vi "Calibration Scaling (Set).vi"(6 "ISOBUS address":T4=-1 caption="ISOBUS address (-1)", 8 "error in":errorcluster, 9 "Unit":T1, 10 "Scaling Factor":dbl=0.5 min=0.5 max=1.5 step=0.1, 11 "Mercury Reference In":T5) -> (0 "error out":errorcluster, 2 "Response":T2, 3 "Mercury Reference Out":T5, 4 "Valid?":T3)   [LabVIEW 2015, in "Mercury iXX.lvlib" / "Pressure.lvlib"]
doc: "Set the current value of the pressure scaling factor."
uses:
  Pressure.lvlib
  Controls/Mercury Reference.ctl
  Controls/Comms Transport Layer.ctl
  private/Controls/Query Dynamic Reference.ctl
  Controls/ISOBus Address.ctl
  Controls/Is Valid LED.ctl
  Controls/Response String.ctl
  Controls/Unit String.ctl
  private/Controls/Command Verbs.ctl
  Mercury iXX.lvlib
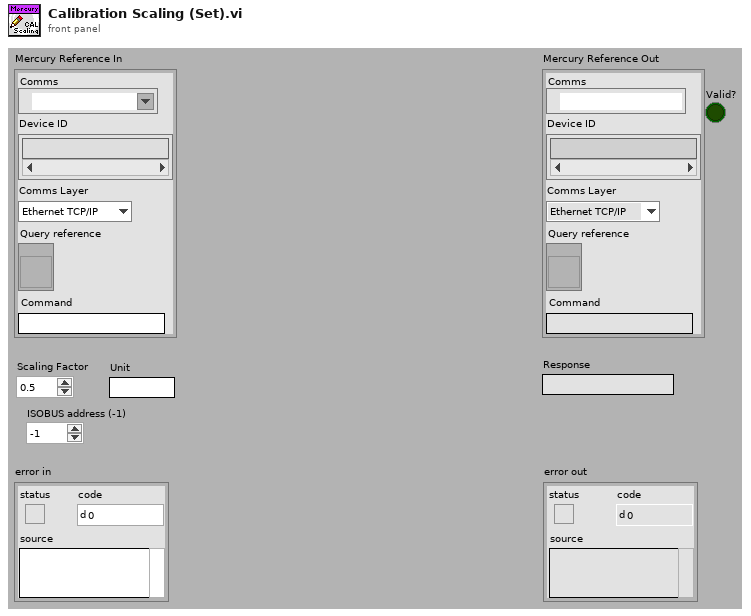
[diagram p1: front panel]
types:
  T1 = typedef "Mercury iXX.lvlib/Unit String.ctl" = string
  T2 = typedef "Mercury iXX.lvlib/Response String.ctl" = string
  T3 = typedef "Mercury iXX.lvlib/Is Valid LED.ctl" = bool
  T4 = typedef "Mercury iXX.lvlib/ISOBus Address.ctl" = i32
  T5 = typedef "Mercury iXX.lvlib/Mercury Reference.ctl" = cluster{"Comms":refnum<visa-resource-name>, "Device ID":string[], "Comms Layer":T6, "Command":string, "Query reference":T7}
  T6 = typedef "Mercury iXX.lvlib/Comms Transport Layer.ctl" = enum16{"Ethernet TCP/IP", "USB", "ISOBus - RS-232", "GPIB"}
  T7 = typedef "Mercury iXX.lvlib/Query Dynamic Reference.ctl" = refnum<vi>
  T8 = typedef "Mercury iXX.lvlib/Command Verbs.ctl" = string
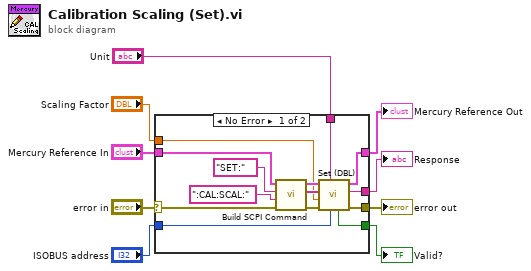
[diagram p0: block diagram]
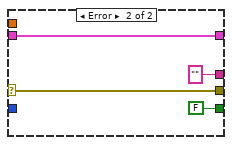
[diagram p2: hidden frame]
diagram:
  n1 = case shown="No Error" "error in" {
    selector: "error in" -> [w11 w27]
    tunnel: "Mercury Reference In" -> [w18 w26]
    tunnel: "Scaling Factor" -> [w17 _]
    tunnel: [w16 w26] -> w7
    tunnel: [w15 T2 "" ("Response")] -> w6
    tunnel: [w14 T3 FALSE ("Valid?")] -> w5
    tunnel: [w13 w27] -> w4
    tunnel: "ISOBUS address" -> [w12 _]
    tunnel: "Unit" -> [w10 _]
    frame No Error {
      n2 = call "Build SCPI Command.vi"("error in"=w11, "Noun(s)"=":CAL:SCAL:" ("Command"), "Verb"=T8 "SET:", "Mercury Reference In"=w18) -> ("error out"=w20:errorcluster, "SCPI Message(s)"=w21:string[], "Mercury Reference Out"=w22:T5)  [unwired: 5 out]
      n3 = call "Set (DBL).vi"("ISOBUS address"=w12, "Unit"=w10, "error in"=w20, "Command Value (Dbl)"=w17, "SCPI Message(s)"=w21, "Mercury Reference In"=w22) -> ("error out"=w13:errorcluster, "Response"=w15:T2, "Mercury Reference Out"=w16:T5, "Valid?"=w14:T3)  [unwired: 2 out]
    }
    frame Error {
    }
  }
  "Mercury Reference Out" <- w7
  "error out" <- w4
  "Valid?" <- w5
  "Response" <- w6
